vi "Begin.vi"(11 "Image Size":T1=enum."160x120") -> (0 "error out":errorcluster)   [LabVIEW 2012]
doc: "Called before other user functions, this VI is expected to open initial I/O refnums, load in file data, and do all program initialization. Notice that the <B>error out</B> terminal is simply used for data flow. Wiring it to other structures or subVIs ensures that this VI runs first."
uses:
  <vilib>/Rock Robotics/WPI/Camera/WPI_CameraImageSize.ctl
  <vilib>/Rock Robotics/SystemInterfaces/DIO/FPGA_DIOPWMChannel.ctl
  <vilib>/Rock Robotics/WPI/Joystick/WPI_JoystickDeviceEnum.ctl
  <vilib>/Rock Robotics/WPI/Camera/WPI_CameraWhite Balance Values.ctl
  <vilib>/Rock Robotics/WPI/Camera/WPI_CameraExposure Values.ctl
  <vilib>/Rock Robotics/WPI/Camera/WPI_CameraFrameRate.ctl
  <vilib>/Rock Robotics/SystemInterfaces/DIO/FPGA_DIOChannel.ctl
  <vilib>/Rock Robotics/SystemInterfaces/Typedef/FPGA_TypedefDigitalModule.ctl
  <vilib>/Rock Robotics/WPI/Encoder/WPI_EncoderType.ctl
  <vilib>/Rock Robotics/SystemInterfaces/DIO/FPGA_DIORelayChannel.ctl
  <vilib>/Rock Robotics/SystemInterfaces/Typedef/FPGA_TypedefAnalogModuleForGyro.ctl
  <vilib>/Rock Robotics/SystemInterfaces/AI/FPGA_AIGyroChannel.ctl
  <vilib>/Rock Robotics/WPI/Relay/WPI_RelayDirection.ctl
  <vilib>/Rock Robotics/WPI/MotorControl/WPI_MotorControlOpen Victor.vi
  <vilib>/Rock Robotics/WPI/RobotDrive/WPI_RobotDriveOpen4MotorWithJaguar.vi
  Robot Global Data.vi
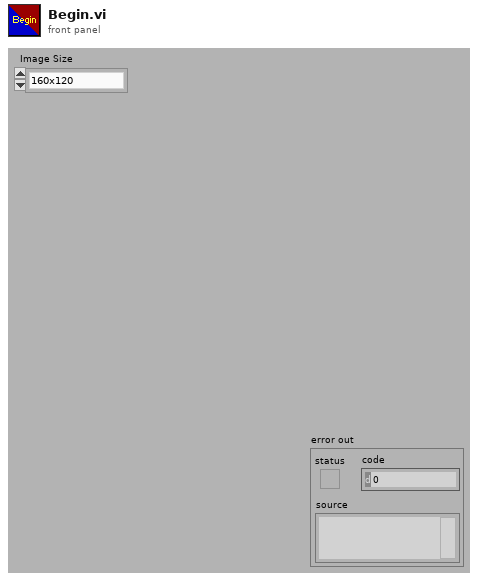
[diagram p1: front panel]
types:
  T1 = typedef "WPI_CameraImageSize.ctl" = enum16{"640x480", "320x240", "160x120"}
  T2 = typedef "FPGA_DIOChannel.ctl" = enum8{"DIO 1", "DIO 2", "DIO 3", "DIO 4", "DIO 5", "DIO 6", "DIO 7", "DIO 8", "DIO 9", "DIO 10", "DIO 11", "DIO 12", "DIO 13", "DIO 14", "Invalid"}
  T3 = typedef "WPI_EncoderType.ctl" = enum16{"1x", "2x", "4x"}
  T4 = typedef "WPI_RelayDirection.ctl" = enum16{"Both directions", "Forward only", "Reverse only"}
  T5 = typedef "FPGA_TypedefDigitalModule.ctl" = enum16{"Digital Module 1", "Digital Module 2"}
  T6 = typedef "FPGA_AIGyroChannel.ctl" = enum8{"AI 1", "AI 2", "Invalid"}
  T7 = typedef "FPGA_TypedefAnalogModuleForGyro.ctl" = enum16{"Analog Module 1"}
  T8 = typedef "FPGA_DIORelayChannel.ctl" = enum8{"Relay 1", "Relay 2", "Relay 3", "Relay 4", "Relay 5", "Relay 6", "Relay 7", "Relay 8", "Invalid"}
  T9 = typedef "FPGA_DIOPWMChannel.ctl" = enum8{"PWM 1", "PWM 2", "PWM 3", "PWM 4", "PWM 5", "PWM 6", "PWM 7", "PWM 8", "PWM 9", "PWM 10", "Invalid"}
  T10 = typedef "WPI_JoystickDeviceEnum.ctl" = enum16{"USB 1", "USB 2", "USB 3", "USB 4", "Kinect 1", "Kinect 2"}
  T11 = typedef "WPI_CameraFrameRate.ctl" = u32
  T12 = typedef "WPI_CameraExposure Values.ctl" = enum16{"Auto", "Flicker-free 50 Hz", "Flicker-free 60 Hz", "Hold current"}
  T13 = typedef "WPI_CameraWhite Balance Values.ctl" = enum16{"Auto", "Fixed indoor", "Fixed outdoor 1", "Fixed outdoor 2", "Fixed fluorescent 1", "Fixed fluorescent 2", "Hold current"}
  T14 = typedef "WPI_CameraDevRef.ctl" = cluster{"Camera Address":string, "CameraStatus":errorcluster, "Acquire Image Notifier":refnum<notifier>}
  T15 = typedef "WPI_DigitalInputDevRef.ctl" = cluster{"DevStatus":errorcluster, "DIO Channel":T2, "Digital Module":T5}
  T16 = typedef "FPGA_CounterEncoderSourceConvertionLVSourceType.ctl" = cluster{"DevStatus":errorcluster, "AnalogTriggerMode?":bool, "DigitalMode":cluster{"Digital Module":T5, "DIO Channel":T17}, "AnalogTriggerMode":cluster{"AnalogTriggerIndex":T18, "OutputType":T19}}
  T17 = typedef "FPGA_DIODigitalSourceChannel.ctl" = enum8{"DIO 1", "DIO 2", "DIO 3", "DIO 4", "DIO 5", "DIO 6", "DIO 7", "DIO 8", "DIO 9", "DIO 10", "DIO 11", "DIO 12", "DIO 13", "DIO 14", "Disabled"}
  T18 = typedef "FPGA_AnalogTriggerIndex.ctl" = enum8{"Trig 0", "Trig 1", "Trig 2", "Trig 3", "Trig 4", "Trig 5", "Trig 6", "Trig 7", "Invalid"}
  T19 = typedef "FPGA_AnalogTriggerOutType.ctl" = enum16{"InWindow", "TriggerState", "Rising", "Falling"}
  T20 = typedef "WPI_GyroDevRef.ctl" = cluster{"DevStatus":errorcluster, "Analog Module":T21, "Analog Channel":T22, "Offset":dbl, "Gain (VoltsPerDegree/Second)":dbl}
  T21 = typedef "FPGA_TypedefAnalogModule.ctl" = enum16{"Analog Module 1", "Analog Module 2"}
  T22 = typedef "FPGA_AIChannel.ctl" = enum8{"AI 1", "AI 2", "AI 3", "AI 4", "AI 5", "AI 6", "AI 7", "AI 8", "Invalid"}
  T23 = typedef "WPI_EncoderDevRef.ctl" = cluster{"DevStatus":errorcluster, "EncoderIndex":T24, "CounterIndex":T25, "DistancePerCount":dbl, "Decoding Type":T3}
  T24 = typedef "FPGA_EncoderIdx.ctl" = enum8{"Enc 0", "Enc 1", "Enc 2", "Enc 3", "Invalid"}
  T25 = typedef "FPGA_CounterCtrSystemIndex.ctl" = enum8{"Ctr 0", "Ctr 1", "Ctr 2", "Ctr 3", "Ctr 4", "Ctr 5", "Ctr 6", "Ctr 7", "Invalid"}
  T26 = typedef "WPI_RobotDriveDevRef.ctl" = cluster{"DevStatus":errorcluster, "Motors[]":T27[], "Square Inputs":bool, "Max Output":dbl, "Isochronous":bool}
  T27 = typedef "WPI_MotorControlDeviceRef.ctl" = cluster{"DeviceStatus":errorcluster, "Type":enum16{"PWM", "CAN"}, "PWM":cluster{"Digital Module":T5, "PWM Channel":T9, "DeadBand":T28}, "CAN":cluster{"Device Number":u8, "Control Mode":T29, "Semaphore":T30, "Max Vout":dbl}, "Invert":bool, "TransformRef":T31, "InvTransformRef":T31}
  T28 = typedef "WPI_PWMDeadband.ctl" = cluster{"Name":string, "maxPositivePwm":i32, "minPositivePwm":i32, "centerPwm":i32, "maxNegativePwm":i32, "minNegativePwm":i32, "angularRange":u16}
  T29 = typedef "WPI_CANJaguar_ControlMode.ctl" = enum8{"Percent VBus", "Current", "Speed", "Position", "Voltage"}
  T30 = typedef "Semaphore RefNum" = refnum<k1>
  T31 = typedef "WPI_PWMTransform_ConPane.ctl" = refnum<vi>
  T32 = typedef "WPI_RelayDevRef.ctl" = cluster{"DevStatus":errorcluster, "Relay Channel":T8, "Digital Module":T5, "Relay Direction":T4}
  T33 = typedef "WPI_JoystickDevRef.ctl" = cluster{"Device":T10}
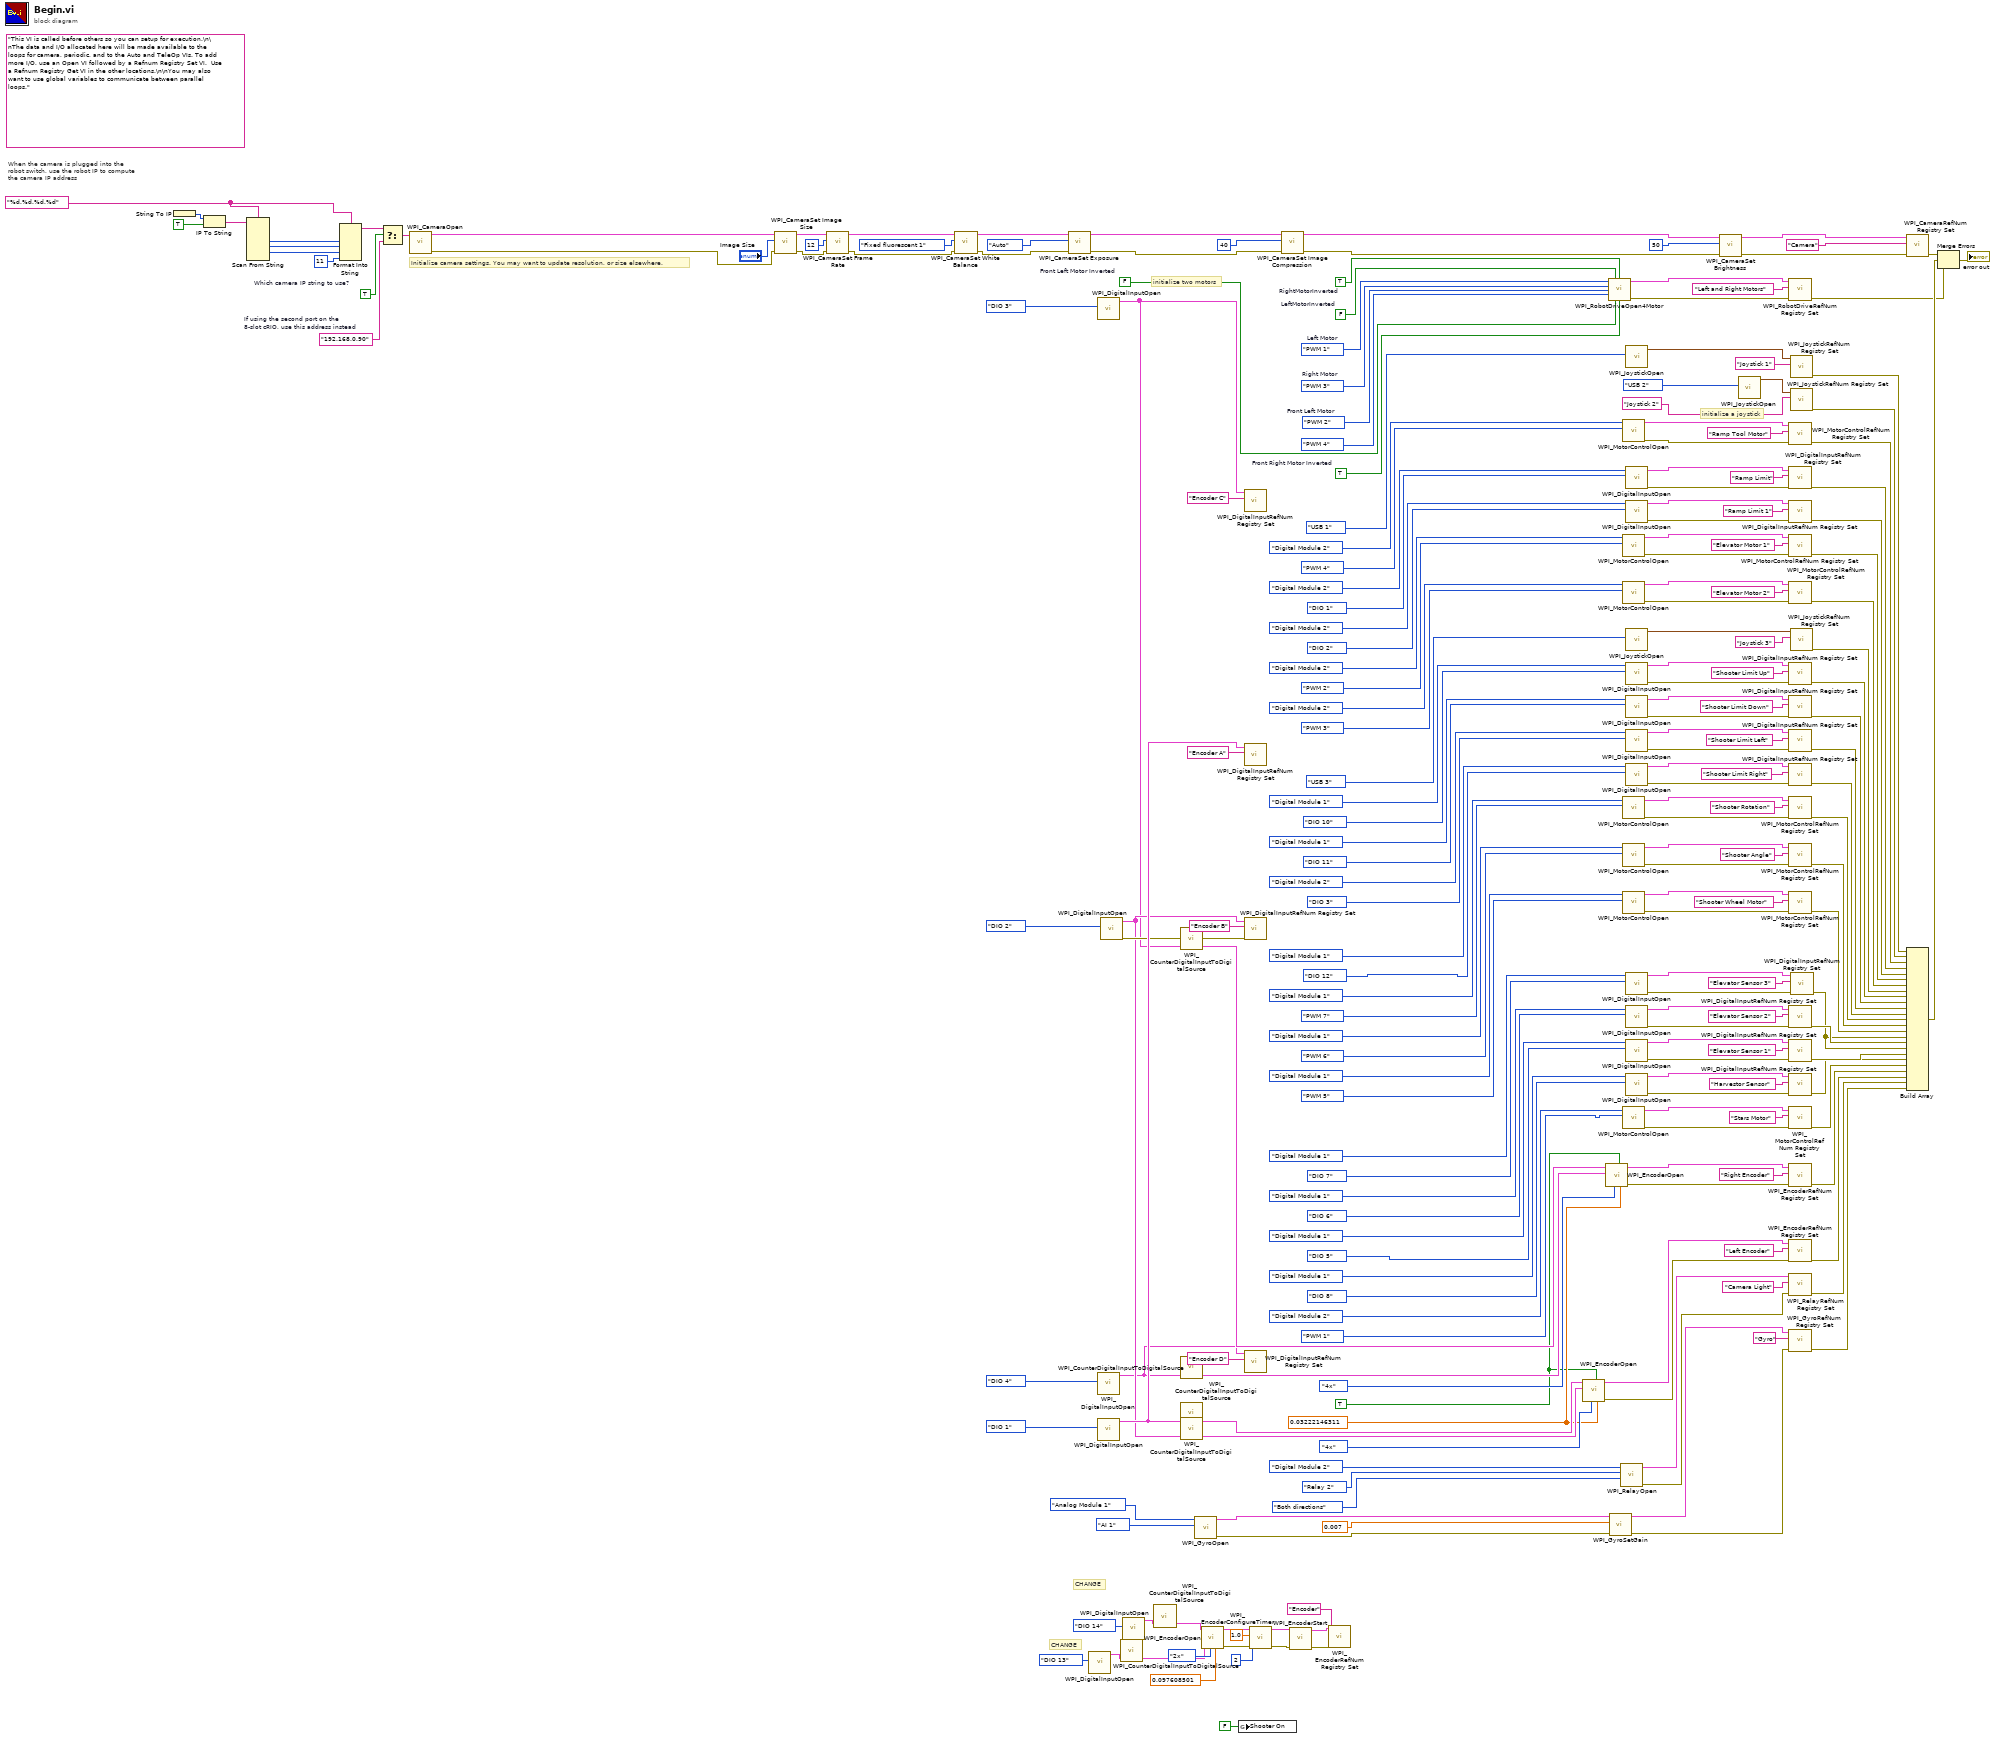
[diagram p0: block diagram]
diagram:
  w27 = FALSE  # Front Left Motor Inverted
  w28 = TRUE  # Front Right Motor Inverted
  w69 = TRUE ("External Reset Active High")
  w79 = 0.03222146311 ("DistancePerCount")
  w165 = FPGA_DIOPWMChannel."PWM 2"  # Front Left Motor
  w183 = TRUE  # Which camera IP string to use?
  w187 = "%d.%d.%d.%d" ("format string")
  (unwired) "This VI is called before others so you can setup for execution.\n\nThe data and I/O allocated here will be made available to the loops for camera, periodic, and to the Auto and TeleOp VIs. To add more I/O, use an Open VI followed by a Refnum Registry Set VI.  Use a Refnum Registry Get VI in the other locations.\n\nYou may also want to use global variables to communicate between parallel loops."
  w199 = FPGA_DIOPWMChannel."PWM 3"  # Right Motor
  w200 = FPGA_DIOPWMChannel."PWM 1"  # Left Motor
  w184 = "192.168.0.90"  # If using the second port on the 8-slot cRIO, use this address instead
  w224 = FALSE  # LeftMotorInverted
  w225 = TRUE  # RightMotorInverted
  # "CHANGE"
  # "CHANGE"
  # "When the camera is plugged into the\nrobot switch, use the robot IP to compute\nthe camera IP address"
  # "initialize a joystick"
  # "initialize two motors"
  # "Initialize camera settings. You may want to update resolution, or size elsewhere."
  n1 = String To IP() -> (0:w194:u32)  [unwired: 1 in]
  n2 = IP To String(1:TRUE ("dot notation? (F)"), 2:w194) -> (0:w192:string)
  n3 = Scan From String(format string=w187, input string=w192) -> (output 1=w191:i32, output 2=w190:i32, output 3=w189:i32)  [unwired: 7 in, 3 out]
  n4 = Format Into String(format string=w187, w191, w190, w189, 11 ("Compression")) -> (resulting string=w185:string)  [unwired: 2 in, 1 out]
  n5 = Select(t=w185, s=w183, f=w184) -> (s? t:f=w186:string)
  n6 = call <vilib>:"WPI_CameraOpen.vi"("Camera Address"=w186) -> ("error out"=w209:errorcluster, "CameraDevRef"=w210:T14)  [unwired: 1 in, 8 out]
  n7 = call <vilib>:"WPI_CameraSet Image Size.vi"("error in (no error)"=w209, "Image Size"="Image Size", "CameraDevRef"=w210) -> ("error out"=w208:errorcluster, "CameraDevRef Out"=w211:T14)  [unwired: 7 out]
  n8 = call <vilib>:"WPI_CameraSet Frame Rate.vi"("error in (no error)"=w208, "Frame Rate (fps)"=T11 12, "CameraDevRef"=w211) -> ("error out"=w207:errorcluster, "CameraDevRef Out"=w213:T14)  [unwired: 7 out]
  n9 = call <vilib>:"WPI_CameraSet White Balance.vi"("error in (no error)"=w207, "White Balance"=WPI_CameraWhite_Balance_Values."Fixed fluorescent 1", "CameraDevRef"=w213) -> ("error out"=w206:errorcluster, "CameraDevRef Out"=w212:T14)  [unwired: 7 out]
  n10 = call <vilib>:"WPI_CameraSet Exposure.vi"("error in (no error)"=w206, "Exposure"=WPI_CameraExposure_Values."Auto", "CameraDevRef"=w212) -> ("error out"=w205:errorcluster, "CameraDevRef Out"=w215:T14)  [unwired: 7 out]
  n11 = call <vilib>:"WPI_DigitalInputOpen.vi"("DIO Channel"=FPGA_DIOChannel."DIO 13") -> ("DigitalInputDevRef"=w3:T15)  [unwired: 9 in, 1 out]
  n12 = call <vilib>:"WPI_DigitalInputOpen.vi"("DIO Channel"=FPGA_DIOChannel."DIO 3") -> ("DigitalInputDevRef"=w73:T15)  [unwired: 2 in, 8 out]
  n13 = call <vilib>:"WPI_DigitalInputOpen.vi"("DIO Channel"=FPGA_DIOChannel."DIO 4") -> ("DigitalInputDevRef"=w72:T15)  [unwired: 2 in, 8 out]
  n14 = call <vilib>:"WPI_DigitalInputOpen.vi"("DIO Channel"=FPGA_DIOChannel."DIO 1") -> ("DigitalInputDevRef"=w78:T15)  [unwired: 2 in, 8 out]
  n15 = call <vilib>:"WPI_DigitalInputOpen.vi"("DIO Channel"=FPGA_DIOChannel."DIO 2") -> ("error out"=w76:errorcluster, "DigitalInputDevRef"=w75:T15)  [unwired: 2 in, 7 out]
  n16 = call <vilib>:"WPI_CounterDigitalInputToDigitalSource.vi"("DigitalInputDevRef"=w3) -> ("Digital Source"=w1:T16)  [unwired: 6 out]
  n17 = call <vilib>:"WPI_DigitalInputOpen.vi"("DIO Channel"=FPGA_DIOChannel."DIO 14") -> ("DigitalInputDevRef"=w10:T15)  [unwired: 9 in, 1 out]
  n18 = call <vilib>:"WPI_CounterDigitalInputToDigitalSource.vi"("DigitalInputDevRef"=w10) -> ("Digital Source"=w9:T16)  [unwired: 6 out]
  n19 = call <vilib>:"WPI_CounterDigitalInputToDigitalSource.vi"("DigitalInputDevRef"=w73) -> ("Digital Source"=w82:T16)  [unwired: 6 out]
  n20 = call <vilib>:"WPI_CounterDigitalInputToDigitalSource.vi"("DigitalInputDevRef"=w72) -> ("Digital Source"=w80:T16)  [unwired: 6 out]
  n21 = call <vilib>:"WPI_CounterDigitalInputToDigitalSource.vi"("DigitalInputDevRef"=w78) -> ("Digital Source"=w86:T16)  [unwired: 6 out]
  n22 = call <vilib>:"WPI_CounterDigitalInputToDigitalSource.vi"("DigitalInputDevRef"=w75) -> ("Digital Source"=w85:T16)  [unwired: 6 out]
  n23 = call <vilib>:"WPI_GyroOpen.vi"("Analog Channel"=FPGA_AIGyroChannel."AI 1", "Analog Module (Module 1)"=FPGA_TypedefAnalogModuleForGyro."Analog Module 1" ("Analog Module (Slot 1)")) -> ("error out"=w33:errorcluster, "GyroDevRef"=w37:T20)  [unwired: 4 in, 4 out]
  n24 = call <vilib>:"WPI_EncoderOpen.vi"("DistancePerCount"=0.097608501, "Decoding Type"=WPI_EncoderType."2x", "BSource"=w1, "ASource"=w9) -> ("error out"=w16:errorcluster, "EncoderDevRef"=w17:T23)  [unwired: 6 in]
  n25 = global write "Robot Global Data.vi" "Shooter On"(FALSE ("Shooter On")) -> ()
  n26 = call <vilib>:"WPI_DigitalInputRefNum Registry Set.vi"("refnum name"="Encoder C", "DigitalInputDevRef"=w73) -> ()  [unwired: 1 in, 9 out]
  n27 = call <vilib>:"WPI_DigitalInputRefNum Registry Set.vi"("refnum name"="Encoder A", "DigitalInputDevRef"=w78) -> ()  [unwired: 1 in, 9 out]
  n28 = call <vilib>:"WPI_DigitalInputRefNum Registry Set.vi"("error in (no error)"=w76, "refnum name"="Encoder B", "DigitalInputDevRef"=w75) -> ()  [unwired: 9 out]
  n29 = call <vilib>:"WPI_DigitalInputRefNum Registry Set.vi"("refnum name"="Encoder D", "DigitalInputDevRef"=w72) -> ()  [unwired: 1 in, 9 out]
  n30 = call <vilib>:"WPI_EncoderConfigureTimer.vi"("error in (no error)"=w16, "Number Samples to Average"=u8 2, "Minimum Rate"=1.0, "EncoderDevRef"=w17) -> ("error out"=w14:errorcluster, "EncoderDevRef"=w15:T23)  [unwired: 6 in]
  n31 = call <vilib>:"WPI_CameraSet Image Compression.vi"("error in (no error)"=w205, "Compression"=40, "CameraDevRef"=w215) -> ("error out"=w204:errorcluster, "CameraDevRef Out"=w214:T14)  [unwired: 7 out]
  n32 = call <vilib>:"WPI_EncoderStart.vi"("error in (no error)"=w14, "EncoderDevRef"=w15) -> ("error out"=w12:errorcluster, "EncoderDevRef"=w13:T23)  [unwired: 8 in]
  n33 = call <vilib>:"WPI_EncoderRefNum Registry Set.vi"("error in (no error)"=w12, "refnum name"="Encoder", "EncoderDevRef"=w13) -> ()  [unwired: 7 in, 2 out]
  n34 = call <vilib>:"WPI_EncoderOpen.vi"("DistancePerCount"=w79, "External Reset Active High"=w69, "Decoding Type"=WPI_EncoderType."4x", "BSource"=w85, "ASource"=w86) -> ("error out"=w94:errorcluster, "EncoderDevRef"=w93:T23)  [unwired: 3 in, 2 out]
  n35 = call <vilib>:"WPI_EncoderOpen.vi"("DistancePerCount"=w79, "External Reset Active High"=w69, "Decoding Type"=WPI_EncoderType."4x", "BSource"=w80, "ASource"=w82) -> ("error out"=w92:errorcluster, "EncoderDevRef"=w91:T23)  [unwired: 3 in, 2 out]
  n36 = call-poly <vilib>:"WPI_RobotDriveOpen4Motor.vi"("Rear Left Motor"=w200, "Rear Left Motor Inverted"=w224, "Rear Right Motor Inverted"=w225, "Rear Right Motor"=w199, "Front Left Motor"=w165, "Front Right Motor"=FPGA_DIOPWMChannel."PWM 4", "Front Left Motor Inverted"=w27, "Front Right Motor Inverted"=w28) -> ("RobotDriveDevRef"=w222:T26, "error out"=w218:errorcluster)  [unwired: 6 in]
  n37 = call <vilib>:"WPI_GyroSetGain.vi"("error in (no error)"=w33, "Gain (VoltsPerDegree/Second)"=0.007, "GyroDevRef"=w37) -> ("error out"=w32:errorcluster, "GyroDevRef"=w34:T20)  [unwired: 7 out]
  n38 = call <vilib>:"WPI_RelayOpen.vi"("Relay Direction"=WPI_RelayDirection."Both directions", "Relay Channel"=FPGA_DIORelayChannel."Relay 2", "Digital Module (Module 1)"=FPGA_TypedefDigitalModule."Digital Module 2") -> ("error out"=w41:errorcluster, "RelayDevRef"=w42:T32)  [unwired: 7 in]
  n39 = call-poly <vilib>:"WPI_MotorControlOpen.vi"("PWM Channel"=FPGA_DIOPWMChannel."PWM 4", "Digital Module (Module 1)"=FPGA_TypedefDigitalModule."Digital Module 2") -> ("error out"=w178:errorcluster, "MotorControlDeviceRef"=w179:T27)  [unwired: 8 in]
  n40 = call-poly <vilib>:"WPI_MotorControlOpen.vi"("PWM Channel"=FPGA_DIOPWMChannel."PWM 2", "Digital Module (Module 1)"=FPGA_TypedefDigitalModule."Digital Module 2") -> ("error out"=w161:errorcluster, "MotorControlDeviceRef"=w163:T27)  [unwired: 8 in]
  n41 = call-poly <vilib>:"WPI_MotorControlOpen.vi"("PWM Channel"=FPGA_DIOPWMChannel."PWM 3", "Digital Module (Module 1)"=FPGA_TypedefDigitalModule."Digital Module 2") -> ("error out"=w158:errorcluster, "MotorControlDeviceRef"=w160:T27)  [unwired: 8 in]
  n42 = call-poly <vilib>:"WPI_MotorControlOpen.vi"("PWM Channel"=FPGA_DIOPWMChannel."PWM 7", "Digital Module (Module 1)"=FPGA_TypedefDigitalModule."Digital Module 1") -> ("error out"=w134:errorcluster, "MotorControlDeviceRef"=w135:T27)  [unwired: 8 in]
  n43 = call-poly <vilib>:"WPI_MotorControlOpen.vi"("PWM Channel"=FPGA_DIOPWMChannel."PWM 6", "Digital Module (Module 1)"=FPGA_TypedefDigitalModule."Digital Module 1") -> ("error out"=w129:errorcluster, "MotorControlDeviceRef"=w130:T27)  [unwired: 8 in]
  n44 = call-poly <vilib>:"WPI_MotorControlOpen.vi"("PWM Channel"=FPGA_DIOPWMChannel."PWM 5", "Digital Module (Module 1)"=FPGA_TypedefDigitalModule."Digital Module 1") -> ("error out"=w125:errorcluster, "MotorControlDeviceRef"=w126:T27)  [unwired: 8 in]
  n45 = call-poly <vilib>:"WPI_MotorControlOpen.vi"("PWM Channel"=FPGA_DIOPWMChannel."PWM 1", "Digital Module (Module 1)"=FPGA_TypedefDigitalModule."Digital Module 2") -> ("error out"=w97:errorcluster, "MotorControlDeviceRef"=w98:T27)  [unwired: 8 in]
  n46 = call <vilib>:"WPI_JoystickOpen.vi"("JoystickDevice"=WPI_JoystickDeviceEnum."USB 1") -> ("JoystickDevRef"=w220:T33)  [unwired: 10 out]
  n47 = call <vilib>:"WPI_DigitalInputOpen.vi"("DIO Channel"=FPGA_DIOChannel."DIO 1", "Digital Module (Module 1)"=FPGA_TypedefDigitalModule."Digital Module 2") -> ("error out"=w174:errorcluster, "DigitalInputDevRef"=w173:T15)  [unwired: 8 in]
  n48 = call <vilib>:"WPI_DigitalInputOpen.vi"("DIO Channel"=FPGA_DIOChannel."DIO 2", "Digital Module (Module 1)"=FPGA_TypedefDigitalModule."Digital Module 2") -> ("error out"=w170:errorcluster, "DigitalInputDevRef"=w169:T15)  [unwired: 8 in]
  n49 = call <vilib>:"WPI_JoystickOpen.vi"("JoystickDevice"=WPI_JoystickDeviceEnum."USB 3") -> ("JoystickDevRef"=w153:T33)  [unwired: 10 out]
  n50 = call <vilib>:"WPI_DigitalInputOpen.vi"("DIO Channel"=FPGA_DIOChannel."DIO 10", "Digital Module (Module 1)"=FPGA_TypedefDigitalModule."Digital Module 1") -> ("error out"=w117:errorcluster, "DigitalInputDevRef"=w150:T15)  [unwired: 8 in]
  n51 = call <vilib>:"WPI_DigitalInputOpen.vi"("DIO Channel"=FPGA_DIOChannel."DIO 11", "Digital Module (Module 1)"=FPGA_TypedefDigitalModule."Digital Module 1") -> ("error out"=w116:errorcluster, "DigitalInputDevRef"=w146:T15)  [unwired: 8 in]
  n52 = call <vilib>:"WPI_DigitalInputOpen.vi"("DIO Channel"=FPGA_DIOChannel."DIO 3", "Digital Module (Module 1)"=FPGA_TypedefDigitalModule."Digital Module 2") -> ("error out"=w115:errorcluster, "DigitalInputDevRef"=w142:T15)  [unwired: 8 in]
  n53 = call <vilib>:"WPI_DigitalInputOpen.vi"("DIO Channel"=FPGA_DIOChannel."DIO 12", "Digital Module (Module 1)"=FPGA_TypedefDigitalModule."Digital Module 1") -> ("error out"=w114:errorcluster, "DigitalInputDevRef"=w138:T15)  [unwired: 8 in]
  n54 = call <vilib>:"WPI_DigitalInputOpen.vi"("DIO Channel"=FPGA_DIOChannel."DIO 7", "Digital Module (Module 1)"=FPGA_TypedefDigitalModule."Digital Module 1") -> ("error out"=w113:errorcluster, "DigitalInputDevRef"=w121:T15)  [unwired: 8 in]
  n55 = call <vilib>:"WPI_DigitalInputOpen.vi"("DIO Channel"=FPGA_DIOChannel."DIO 6", "Digital Module (Module 1)"=FPGA_TypedefDigitalModule."Digital Module 1") -> ("error out"=w108:errorcluster, "DigitalInputDevRef"=w112:T15)  [unwired: 8 in]
  n56 = call <vilib>:"WPI_DigitalInputOpen.vi"("DIO Channel"=FPGA_DIOChannel."DIO 5", "Digital Module (Module 1)"=FPGA_TypedefDigitalModule."Digital Module 1") -> ("error out"=w104:errorcluster, "DigitalInputDevRef"=w107:T15)  [unwired: 8 in]
  n57 = call <vilib>:"WPI_DigitalInputOpen.vi"("DIO Channel"=FPGA_DIOChannel."DIO 8", "Digital Module (Module 1)"=FPGA_TypedefDigitalModule."Digital Module 1") -> ("error out"=w99:errorcluster, "DigitalInputDevRef"=w103:T15)  [unwired: 8 in]
  n58 = call <vilib>:"WPI_CameraSet Brightness.vi"("error in (no error)"=w204, "Brightness"=50, "CameraDevRef"=w214) -> ("error out"=w202:errorcluster, "CameraDevRef Out"=w203:T14)  [unwired: 7 out]
  n59 = call <vilib>:"WPI_JoystickOpen.vi"("JoystickDevice"=WPI_JoystickDeviceEnum."USB 2") -> ("JoystickDevRef"=w182:T33)  [unwired: 10 in]
  n60 = call <vilib>:"WPI_RobotDriveRefNum Registry Set.vi"("error in (no error)"=w218, "refnum name"="Left and Right Motors", "RobotDriveDevRef"=w222) -> ("error out"=w19:errorcluster)  [unwired: 8 out]
  n61 = call <vilib>:"WPI_MotorControlRefNum Registry Set.vi"("error in (no error)"=w178, "refnum name"="Ramp Tool Motor", "MotorControlDevRef"=w179) -> ("error out"=w65:errorcluster)  [unwired: 7 in, 1 out]
  n62 = call <vilib>:"WPI_DigitalInputRefNum Registry Set.vi"("error in (no error)"=w174, "refnum name"="Ramp Limit", "DigitalInputDevRef"=w173) -> ("error out"=w64:errorcluster)  [unwired: 7 in, 1 out]
  n63 = call <vilib>:"WPI_DigitalInputRefNum Registry Set.vi"("error in (no error)"=w170, "refnum name"="Ramp Limit 1", "DigitalInputDevRef"=w169) -> ("error out"=w63:errorcluster)  [unwired: 7 in, 1 out]
  n64 = call <vilib>:"WPI_MotorControlRefNum Registry Set.vi"("error in (no error)"=w161, "refnum name"="Elevator Motor 1", "MotorControlDevRef"=w163) -> ("error out"=w62:errorcluster)  [unwired: 7 in, 1 out]
  n65 = call <vilib>:"WPI_MotorControlRefNum Registry Set.vi"("error in (no error)"=w158, "refnum name"="Elevator Motor 2", "MotorControlDevRef"=w160) -> ("error out"=w61:errorcluster)  [unwired: 7 in, 1 out]
  n66 = call <vilib>:"WPI_DigitalInputRefNum Registry Set.vi"("error in (no error)"=w117, "refnum name"="Shooter Limit Up", "DigitalInputDevRef"=w150) -> ("error out"=w59:errorcluster)  [unwired: 7 in, 1 out]
  n67 = call <vilib>:"WPI_DigitalInputRefNum Registry Set.vi"("error in (no error)"=w116, "refnum name"="Shooter Limit Down", "DigitalInputDevRef"=w146) -> ("error out"=w58:errorcluster)  [unwired: 7 in, 1 out]
  n68 = call <vilib>:"WPI_DigitalInputRefNum Registry Set.vi"("error in (no error)"=w115, "refnum name"="Shooter Limit Left", "DigitalInputDevRef"=w142) -> ("error out"=w57:errorcluster)  [unwired: 7 in, 1 out]
  n69 = call <vilib>:"WPI_DigitalInputRefNum Registry Set.vi"("error in (no error)"=w114, "refnum name"="Shooter Limit Right", "DigitalInputDevRef"=w138) -> ("error out"=w56:errorcluster)  [unwired: 7 in, 1 out]
  n70 = call <vilib>:"WPI_MotorControlRefNum Registry Set.vi"("error in (no error)"=w134, "refnum name"="Shooter Rotation", "MotorControlDevRef"=w135) -> ("error out"=w55:errorcluster)  [unwired: 7 in, 1 out]
  n71 = call <vilib>:"WPI_MotorControlRefNum Registry Set.vi"("error in (no error)"=w129, "refnum name"="Shooter Angle", "MotorControlDevRef"=w130) -> ("error out"=w54:errorcluster)  [unwired: 7 in, 1 out]
  n72 = call <vilib>:"WPI_MotorControlRefNum Registry Set.vi"("error in (no error)"=w125, "refnum name"="Shooter Wheel Motor", "MotorControlDevRef"=w126) -> ("error out"=w53:errorcluster)  [unwired: 7 in, 1 out]
  n73 = call <vilib>:"WPI_DigitalInputRefNum Registry Set.vi"("error in (no error)"=w108, "refnum name"="Elevator Sensor 2", "DigitalInputDevRef"=w112) -> ("error out"=w52:errorcluster)  [unwired: 7 in, 1 out]
  n74 = call <vilib>:"WPI_DigitalInputRefNum Registry Set.vi"("error in (no error)"=w104, "refnum name"="Elevator Sensor 1", "DigitalInputDevRef"=w107) -> ("error out"=w50:errorcluster)  [unwired: 7 in, 1 out]
  n75 = call <vilib>:"WPI_DigitalInputRefNum Registry Set.vi"("error in (no error)"=w99, "refnum name"="Harvestor Sensor", "DigitalInputDevRef"=w103) -> ("error out"=w49:errorcluster)  [unwired: 7 in, 1 out]
  n76 = call <vilib>:"WPI_MotorControlRefNum Registry Set.vi"("error in (no error)"=w97, "refnum name"="Stars Motor", "MotorControlDevRef"=w98) -> ("error out"=w48:errorcluster)  [unwired: 7 in, 1 out]
  n77 = call <vilib>:"WPI_EncoderRefNum Registry Set.vi"("error in (no error)"=w92, "refnum name"="Right Encoder", "EncoderDevRef"=w91) -> ("error out"=w47:errorcluster)  [unwired: 8 out]
  n78 = call <vilib>:"WPI_EncoderRefNum Registry Set.vi"("error in (no error)"=w94, "refnum name"="Left Encoder", "EncoderDevRef"=w93) -> ("error out"=w46:errorcluster)  [unwired: 8 out]
  n79 = call <vilib>:"WPI_RelayRefNum Registry Set.vi"("error in (no error)"=w41, "refnum name"="Camera Light", "RelayDevRef"=w42) -> ("error out"=w38:errorcluster)  [unwired: 7 in, 1 out]
  n80 = call <vilib>:"WPI_GyroRefNum Registry Set.vi"("error in (no error)"=w32, "refnum name"="Gyro", "GyroDevRef"=w34) -> ("error out"=w29:errorcluster)  [unwired: 8 out]
  n81 = call <vilib>:"WPI_JoystickRefNum Registry Set.vi"("refnum name"="Joystick 1", "JoystickDevRef"=w220) -> ("error out"=w67:errorcluster)  [unwired: 1 in, 8 out]
  n82 = call <vilib>:"WPI_JoystickRefNum Registry Set.vi"("refnum name"="Joystick 2", "JoystickDevRef"=w182) -> ("error out"=w66:errorcluster)  [unwired: 8 in, 1 out]
  n83 = call <vilib>:"WPI_JoystickRefNum Registry Set.vi"("refnum name"="Joystick 3", "JoystickDevRef"=w153) -> ("error out"=w60:errorcluster)  [unwired: 1 in, 8 out]
  n84 = call <vilib>:"WPI_DigitalInputRefNum Registry Set.vi"("error in (no error)"=w113, "refnum name"="Elevator Sensor 3", "DigitalInputDevRef"=w121) -> ("error out"=w51:errorcluster)  [unwired: 7 in, 1 out]
  n85 = call <vilib>:"WPI_CameraRefNum Registry Set.vi"("error in (no error)"=w202, "refnum name"="Camera", "CameraDevRef"=w203) -> ("error out"=w43:errorcluster)  [unwired: 8 out]
  n86 = Build Array(w67, w66, w65, w64, w63, w62, w61, w60, w59, w58, w57, w56, w55, w54, w53, w51, w52, w51, w50, w49, w48, w47, w46, w38, w29) -> (w44:errorcluster[])
  n87 = Merge Errors(w43, w44, w19) -> (→"error out":errorcluster)
